vi "Open Hardware.vi"(8 "error in (no error)":errorcluster, 11 "Instrument in":refnum<class "Instrument.lvclass">) -> (0 "error out":errorcluster, 3 "Instrument out":refnum<class "Instrument.lvclass">)   [LabVIEW 2019, in "Instrument.lvlib" / "Instrument.lvclass"]
doc: "Override to <b>open</b> a connection to your instrument."
uses:
  Instrument.lvclass
  Instrument.lvclass/Instrument.ctl
  subsystems/HAL/HAL.lvclass
  <vilib>/ErrorRing/Error Ring.xnode
  <vilib>/Utility/error.llb/Error Cluster From Error Code.vi
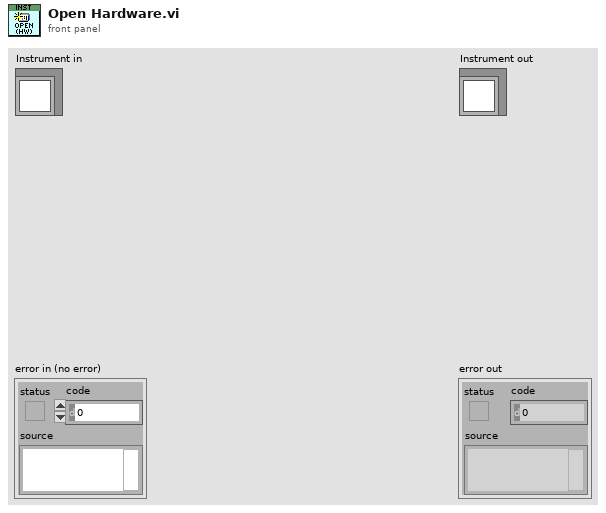
[diagram p1: front panel]
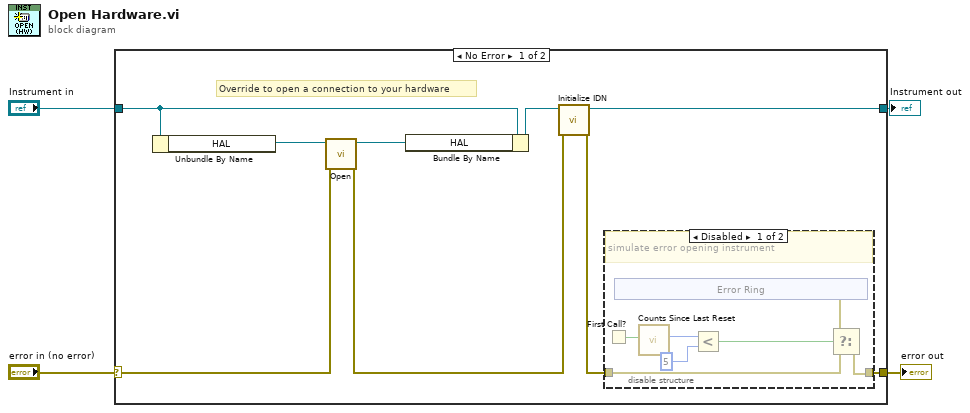
[diagram p0: block diagram]
diagram:
  n1 = case shown="No Error" "error in (no error)" {
    selector: "error in (no error)" -> [w11 w27]
    tunnel: [w13 w27] -> w3
    tunnel: [w7 w26] -> w1
    tunnel: "Instrument in" -> [w10 w26]
    frame No Error {
      # "Override to open a connection to your hardware"
      n2 = Unbundle By Name(w10) -> ("HAL"=w12:refnum<class "HAL.lvclass">)
      n3 = call-dynamic "Open.vi"("error in (no error)"=w11, "HAL in"=w12) -> ("error out"=w6:errorcluster, "HAL out"=w9:refnum<class "HAL.lvclass">)  [unwired: 8 in]
      n4 = Bundle By Name(cluster=w10, "HAL"=w9) -> (w8:refnum<class "Instrument.lvclass">)
      n5 = call "Initialize IDN.vi"("error in (no error)"=w6, "Instrument in"=w8) -> ("error out"=w5:errorcluster, "Instrument out"=w7:refnum<class "Instrument.lvclass">)  [unwired: 8 in]
      n6 = disable-structure shown="Disabled" {
        disable-tunnel: w5 -> [w19 w25]
        disable-tunnel: [w18 w25] -> w13
        frame Disabled {
          # "simulate error opening instrument"
          n7 = First Call?() -> (First Call?: T/F=w16:bool)
          n8 = xnode "Error Ring"() -> ("error out"=w14:errorcluster)
          n9 = call "Counts Since Last Reset.vi"("Reset (F)"=w16) -> ("counter"=w15:u32)  [unwired: 5 in, 1 out]
          n10 = Less?(x=w15, y=u32 5 ("x")) -> (x < y?=w20:bool)
          n11 = Select(t=w14, s=w20, f=w19) -> (s? t:f=w18:errorcluster)
        }
        frame Enabled {
        }
      }
    }
    frame Error {
    }
  }
  "error out" <- w3
  "Instrument out" <- w1
